vi "WriteRead_(SubVI).vi"(8 "error in":errorcluster, 9 "Запрос":string, 11 "ParamIn":T1={"ReadIntParam"=TRUE, "ReadDescrParam"=FALSE, "ReadFloatParam"=TRUE, "debug"=FALSE, "ReadJSON"=TRUE, "IP_address"="192.168.1.216", "N_attempts"=3, "type_con"=enum."TCP", "MB_address"=1, "VISA"="COM1", "connection ID"=refnum, "nameDevices"="", "timeout"=0, "port"=0, "type_version"="0F0C0001", "baud_rate"=115200, "VersionControl"=TRUE, "TCP_conn"=TRUE, "WindowSize"=700}) -> (0 "error out":errorcluster, 2 "Ответ":string, 3 "ParamOut":T1={"ReadIntParam"=TRUE, "ReadDescrParam"=FALSE, "ReadFloatParam"=TRUE, "debug"=FALSE, "ReadJSON"=TRUE, "IP_address"="192.168.1.216", "N_attempts"=3, "type_con"=enum."TCP", "MB_address"=1, "VISA"="COM1", "connection ID"=refnum, "nameDevices"="", "timeout"=0, "port"=0, "type_version"="0F0C0001", "baud_rate"=115200, "VersionControl"=TRUE, "TCP_conn"=TRUE, "WindowSize"=700}, 5 "ErrorMessage":bool, 7 "GatewayTimeout":bool)   [LabVIEW 2017, in "LV_Unicorn.lvlib"]
uses:
  LV_Unicorn.lvlib
  Control/unicorn_conn.ctl
panel:
  out "Attempts":i32
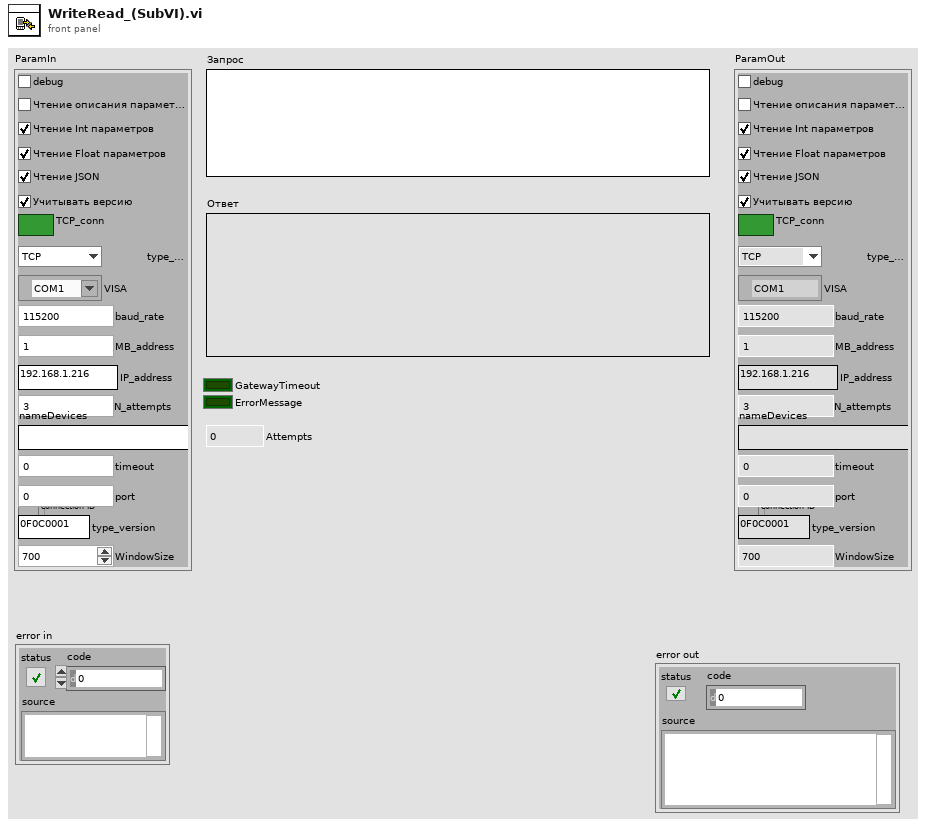
[diagram p1: front panel]
types:
  T1 = typedef "LV_Unicorn.lvlib/unicorn_conn.ctl" = cluster{"ReadIntParam":bool, "ReadDescrParam":bool, "ReadFloatParam":bool, "debug":bool, "ReadJSON":bool, "IP_address":string, "N_attempts":i32, "type_con":enum16{"Serial", "TCP"}, "MB_address":i32, "VISA":refnum<visa-resource-name>, "connection ID":refnum<k5>, "nameDevices":string, "timeout":i32, "port":u16, "type_version":string, "baud_rate":u32, "VersionControl":bool, "TCP_conn":bool, "WindowSize":i32}
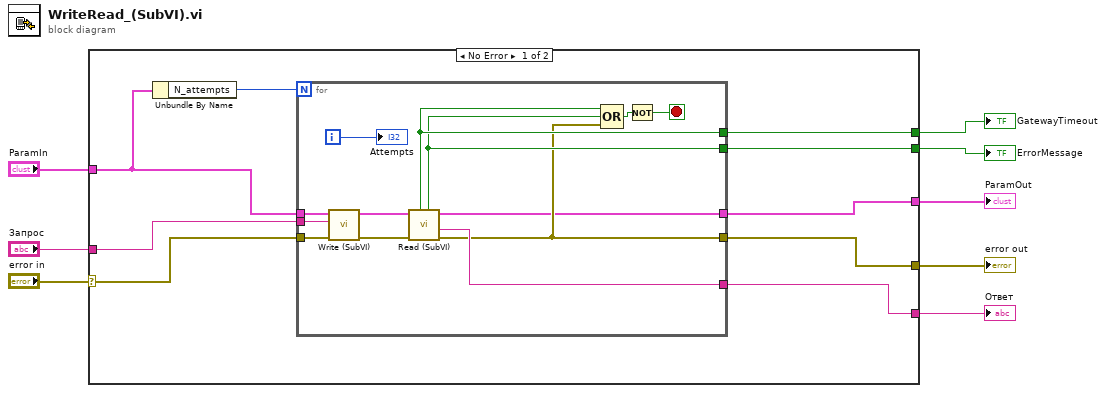
[diagram p0: block diagram]
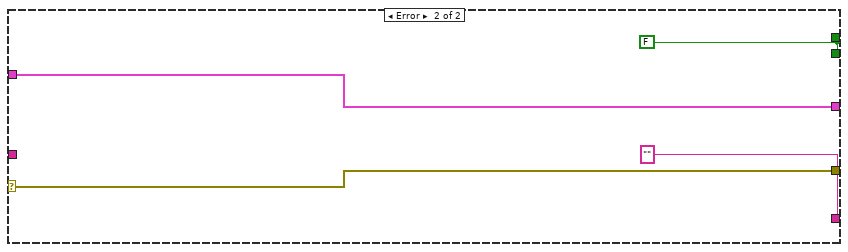
[diagram p2: hidden frame]
diagram:
  n1 = case shown="No Error" "error in" {
    selector: "error in" -> [w11 w34]
    tunnel: "Запрос" -> [w17 _]
    tunnel: [w16 "" ("String out")] -> w7
    tunnel: [w15 w33] -> w6
    tunnel: [w14 w34] -> w5
    tunnel: "ParamIn" -> [w13 w33]
    tunnel: [w10 w31] -> w2
    tunnel: [w9 w31] -> w1
    frame No Error {
      n2 = Unbundle By Name(w13) -> ("N_attempts"=w12:i32)
      n3 = for {
        N: w12 -> [_]
        tunnel: w17 -> [w26]
        tunnel: [w25] -> w16
        tunnel: w13 -> [w27]
        tunnel: [w18] -> w15
        tunnel: w11 -> [w28]
        tunnel: [w19] -> w14
        tunnel: [w21] -> w10
        tunnel: [w20] -> w9
        i -> [w23]
        stop <- w24 stop-if-true
        n4 = call "Write (SubVI).vi"("error in"=w28, "Запрос"=w26, "Param in"=w27) -> ("error out"=w29:errorcluster, "Param out"=w30:T1)  [unwired: 7 in]
        n5 = call "Read (SubVI).vi"("error in (no error)"=w29, "Parameter In"=w30) -> ("error out"=w19:errorcluster, "String out"=w25:string, "Parameter Out"=w18:T1, "ErrorMessage"=w20:bool, "GatewayTimeout"=w21:bool)  [unwired: 5 in]
        n6 = Compound Arithmetic op=OR(w21, w20, w19) -> (w22:bool)
        n7 = Not(x=w22) -> (.not. x?=w24:bool)
        "Attempts" <- w23
      }
    }
    frame Error {
      w31 = FALSE ("Сообщение об ошибке")
    }
  }
  "Ответ" <- w7
  "ParamOut" <- w6
  "error out" <- w5
  "GatewayTimeout" <- w2
  "ErrorMessage" <- w1
